vi "CalculateFit.vi"(8 "X Range":dbl[](array[numeric]), 9 "Response in":dbl[][](array[numeric]), 10 "Stimulus in":dbl[][](array[numeric]), 11 "Mean Fit in":refnum<class "Mean Fit.lvclass">) -> (3 "Mean Fit out":refnum<class "Mean Fit.lvclass">)   [LabVIEW 2016, in "Mean Fit.lvclass"]
uses:
  Mean Fit.lvclass
  Mean Fit.lvclass/Mean Fit.ctl
  comm/nan operations/nan operations.lvlib
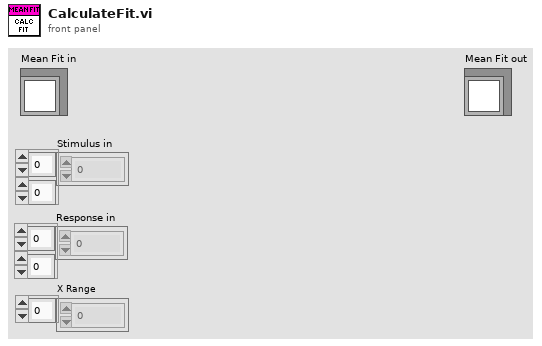
[diagram p1: front panel]
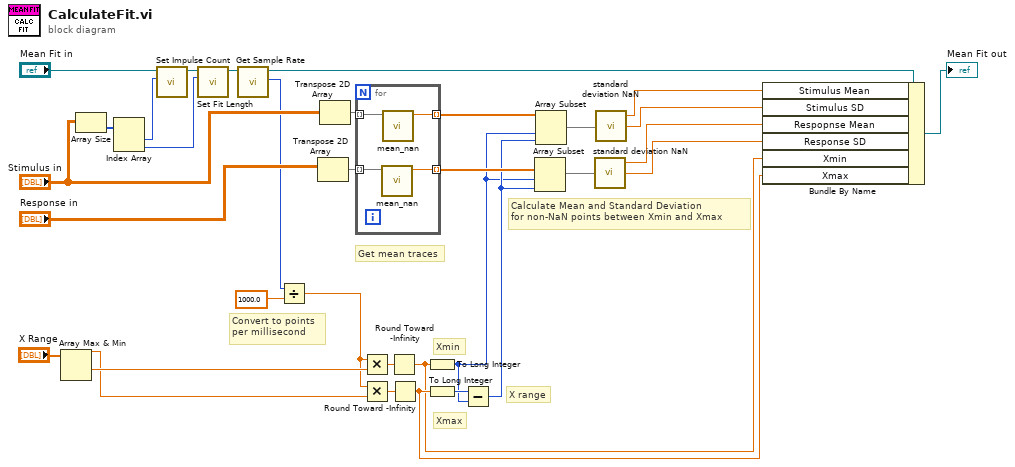
[diagram p0: block diagram]
diagram:
  # "Xmax"
  # "Xmin"
  # "Convert to points\nper millisecond"
  # "X range"
  # "Get mean traces"
  # "Calculate Mean and Standard Deviation\nfor non-NaN points between Xmin and Xmax"
  n1 = Array Max & Min(array="X Range") -> (max value=w4:dbl, min value=w5:dbl)  [unwired: 2 out]
  n2 = Array Size(array="Stimulus in") -> (size(s)=w27:i32[])
  n3 = Index Array(array=w27) -> (element #1=w26:i32, element #2=w11:i32)  [unwired: 2 in]
  n4 = call-dynamic "Set Impulse Count.vi"("Nr of Fit Impulses"=w26, "Abstract Fit in"="Mean Fit in") -> ("Abstract Fit out"=w25:refnum<class "Mean Fit.lvclass">)  [unwired: 8 in, 1 out]
  n5 = call-dynamic "Set Fit Length.vi"("Length"=w11, "Abstract Fit in"=w25) -> ("Abstract Fit out"=w9:refnum<class "Mean Fit.lvclass">)  [unwired: 8 in, 1 out]
  n6 = call-dynamic "Get Sample Rate.vi"("Abstract Fit in"=w9) -> ("Sample Rate"=w2:i32, "Abstract Fit out"=w8:refnum<class "Mean Fit.lvclass">)  [unwired: 8 in, 1 out]
  n7 = Divide(x=w2, y=1000.0) -> (x/y=w1:dbl)
  n8 = Transpose 2D Array(2D array="Response in") -> (transposed array=w22:dbl[][])
  n9 = Transpose 2D Array(2D array="Stimulus in") -> (transposed array=w32:dbl[][])
  n10 = for {
    tunnel: [w37] -> w30 mode=indexing
    tunnel: w32 -> [w36] mode=indexing
    tunnel: w22 -> [w35] mode=indexing
    tunnel: [w34] -> w19 mode=indexing
    n11 = call "mean_nan.vi"("Array"=w35) -> ("Mean"=w34:dbl)  [unwired: 10 in]
    n12 = call "mean_nan.vi"("Array"=w36) -> ("Mean"=w37:dbl)  [unwired: 10 in]
  }
  n13 = Multiply(x=w1, y=w5) -> (x*y=w7:dbl)
  n14 = Multiply(x=w1, y=w4) -> (x*y=w6:dbl)
  n15 = Round Toward -Infinity(1:w7) -> (0:w12:dbl)
  n16 = Round Toward -Infinity(1:w6) -> (0:w13:dbl)
  n17 = To Long Integer(number=w12) -> (32bit integer=w17:i32)
  n18 = To Long Integer(number=w13) -> (32bit integer=w24:i32)
  n19 = Subtract(x=w24, y=w17) -> (x-y=w18:i32)
  n20 = Array Subset(array=w19, index=w17, length=w18) -> (w16:dbl[])
  n21 = Array Subset(array=w30, index=w17, length=w18) -> (w31:dbl[])
  n22 = call "standard deviation NaN.vi"("Array"=w16) -> ("standard deviation"=w14:dbl, "mean"=w15:dbl)  [unwired: 2 in, 1 out]
  n23 = call "standard deviation NaN.vi"("Array"=w31) -> ("standard deviation"=w20:dbl, "mean"=w21:dbl)  [unwired: 2 in, 1 out]
  n24 = Bundle By Name(cluster=w8, "Stimulus Mean"=w21, "Stimulus SD"=w20, "Respopnse Mean"=w15, "Response SD"=w14, "Xmin"=w12, "Xmax"=w13) -> (→"Mean Fit out":refnum<class "Mean Fit.lvclass">)
